vi "Present.vi"(9 "Display Help":bool, 10 "Stats":T1={"Transform And Project Duration"=0.0, "Raster Duration"=0.0, "Present Duration"=82.5692473, "Frame Rate"=111.70812900055276, "Visible Triangles"=0, "Delta Time"=0.0} {"Delta Time" format="%.0p"; "Frame Rate" format="%.0p"; "Present Duration" format="%.0p"; "Raster Duration" format="%.0p"; "Transform And Project Duration" format="%.0p"}, 11 "Pixel Data":u32[][](array[numeric])) -> (2 "Present Duration [s]":dbl format="%.3p", 3 "2D Picture":picture)   [LabVIEW 2022 SP3, in "Application.lvlib"]
uses:
  Application.lvlib
  Scene/Stats.ctl
  5bb89e80-4431-4a04-aab7-f6923ae8e18e.vi
  5002ab1c-b7b6-4038-93be-709e90c08d53.vi
  <vilib>/Utility/High Resolution Relative Seconds.vi
  Libraries/Utility/Convert Seconds To Milliseconds.vi
  <vilib>/picture/picture.llb/Draw Text at Point.vi
  Libraries/Raster/Raster.lvlib
  Scene/Scene.lvclass
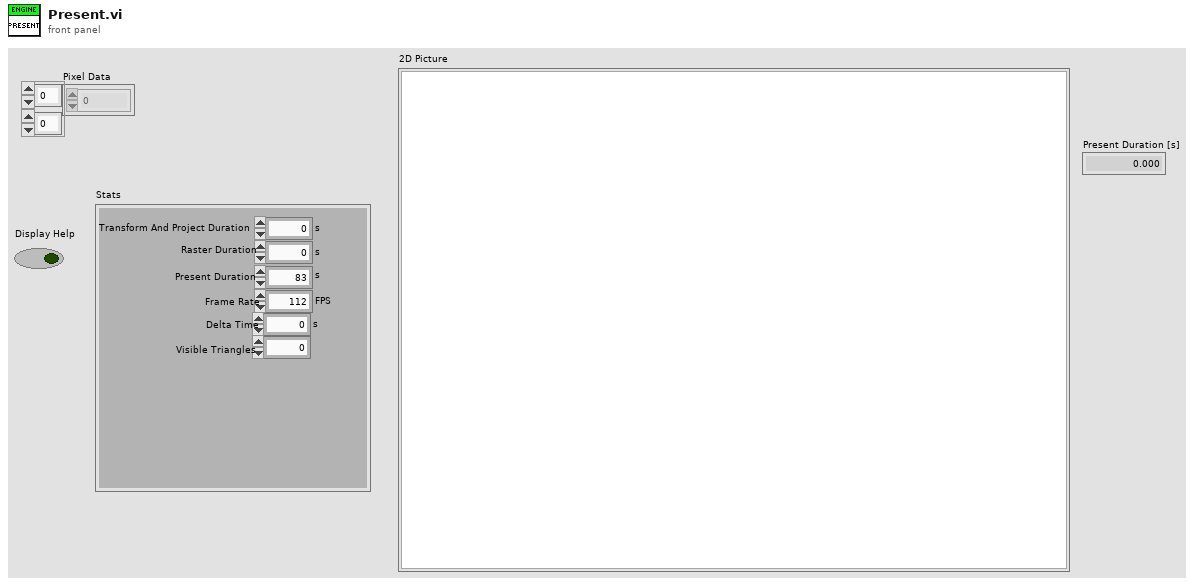
[diagram p1: front panel]
types:
  T1 = typedef "Application.lvlib/Scene.lvclass/Stats.ctl" = cluster{"Transform And Project Duration":dbl, "Raster Duration":dbl, "Present Duration":dbl, "Frame Rate":dbl, "Visible Triangles":i32, "Delta Time":dbl}
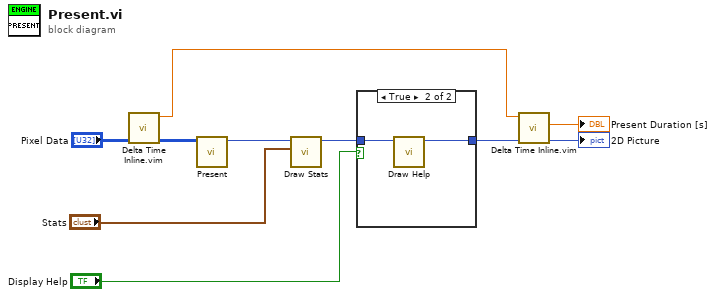
[diagram p0: block diagram]
diagram:
  n1 = call "Delta Time Inline.vim"("value in"="Pixel Data") -> ("value out"=w10:u32[][], "Relative Seconds out [s]"=w2:dbl)  [unwired: 8 in, 1 out]
  n2 = call "Present.vi"("Pixel Data in"=w10) -> ("2D Picture"=w1:picture)  [unwired: 9 in, 1 out]
  n3 = call "Draw Stats.vi"("Stats"="Stats", "Screen in"=w1) -> ("Screen out"=w5:picture)  [unwired: 9 in]
  n4 = case shown="True" "Display Help" {
    tunnel: [w11 w13] -> w6
    tunnel: w5 -> [w11 w12]
    frame False {
    }
    frame True {
      n5 = call "Draw Help.vi"("Screen in"=w12) -> ("Screen out"=w13:picture)  [unwired: 10 in]
    }
  }
  n6 = call "Delta Time Inline.vim"("value in"=w6, "Relative Seconds in [s]"=w2) -> ("value out"=→"2D Picture":picture, "Delta Time [s]"=→"Present Duration [s]":dbl)  [unwired: 7 in, 1 out]
